vi "Watch_SPEC.vi"() -> ()   [LabVIEW 2015]
uses:
  <vilib>/Platform/TimedLoop/XDataNode/timing_clust.ctl
  <vilib>/Platform/TimedLoop/XDataNode/nitl_modes.ctl
  <vilib>/Platform/TimedLoop/XDataNode/wakeup.ctl
  <userlib>/caLab/Private/Get_PV-1D.vi
  <vilib>/platform/TimedLoop/XDataNode/XDataNode.xnode
  <vilib>/Platform/TimedLoop/XDataNode/XDNodeRunTimeDep.lvlib
panel:
  out "EPICS_PVs":string
  in  "Logbook":string(combo)
  out "subarray 2":dbl[](array[numeric])
  out "subarray":dbl[](array[numeric])
  out "XY Graph":cluster{dbl[], dbl[]}(graph)
  out "concatenated string 3":string
  out "standard error 5":string
  out "standard output 5":string
  out "File Name 5":string
  out "x = y? 3":bool
  out "standard output 4":string
  out "standard error 4":string
  out "concatenated string 2":string
  out "spreadsheet string 2":string
  in  "Filter txt":string="*.txt"
  out "File Name 4":string
  out "spreadsheet string 3":string
  out "concatenated string 6":string
  out "standard error 3":string
  out "standard output 3":string
  in  "OK Button":bool
  in  "Maindir":string="P:\\bl13-0\\bl13-2\\dt_SES100\\"
  in  "stop 2":bool
  in  "ELOG":string
  out "path":path
  in  "Subdir":string="2016\\Nilsson\\"
  out "PV Names (dup)":string[](array[string])
  out "PV2ELOG":string
  # "Set a folder to watch using the\nPath control. You can also\nset a filter for a certain type\nof file to watch for (such as\n*.bmp). Then run the\nexample. Whenever you create\na new file in that directory that\nmatches the filter, New File Name\nwill update to let you know the\nnew file name."
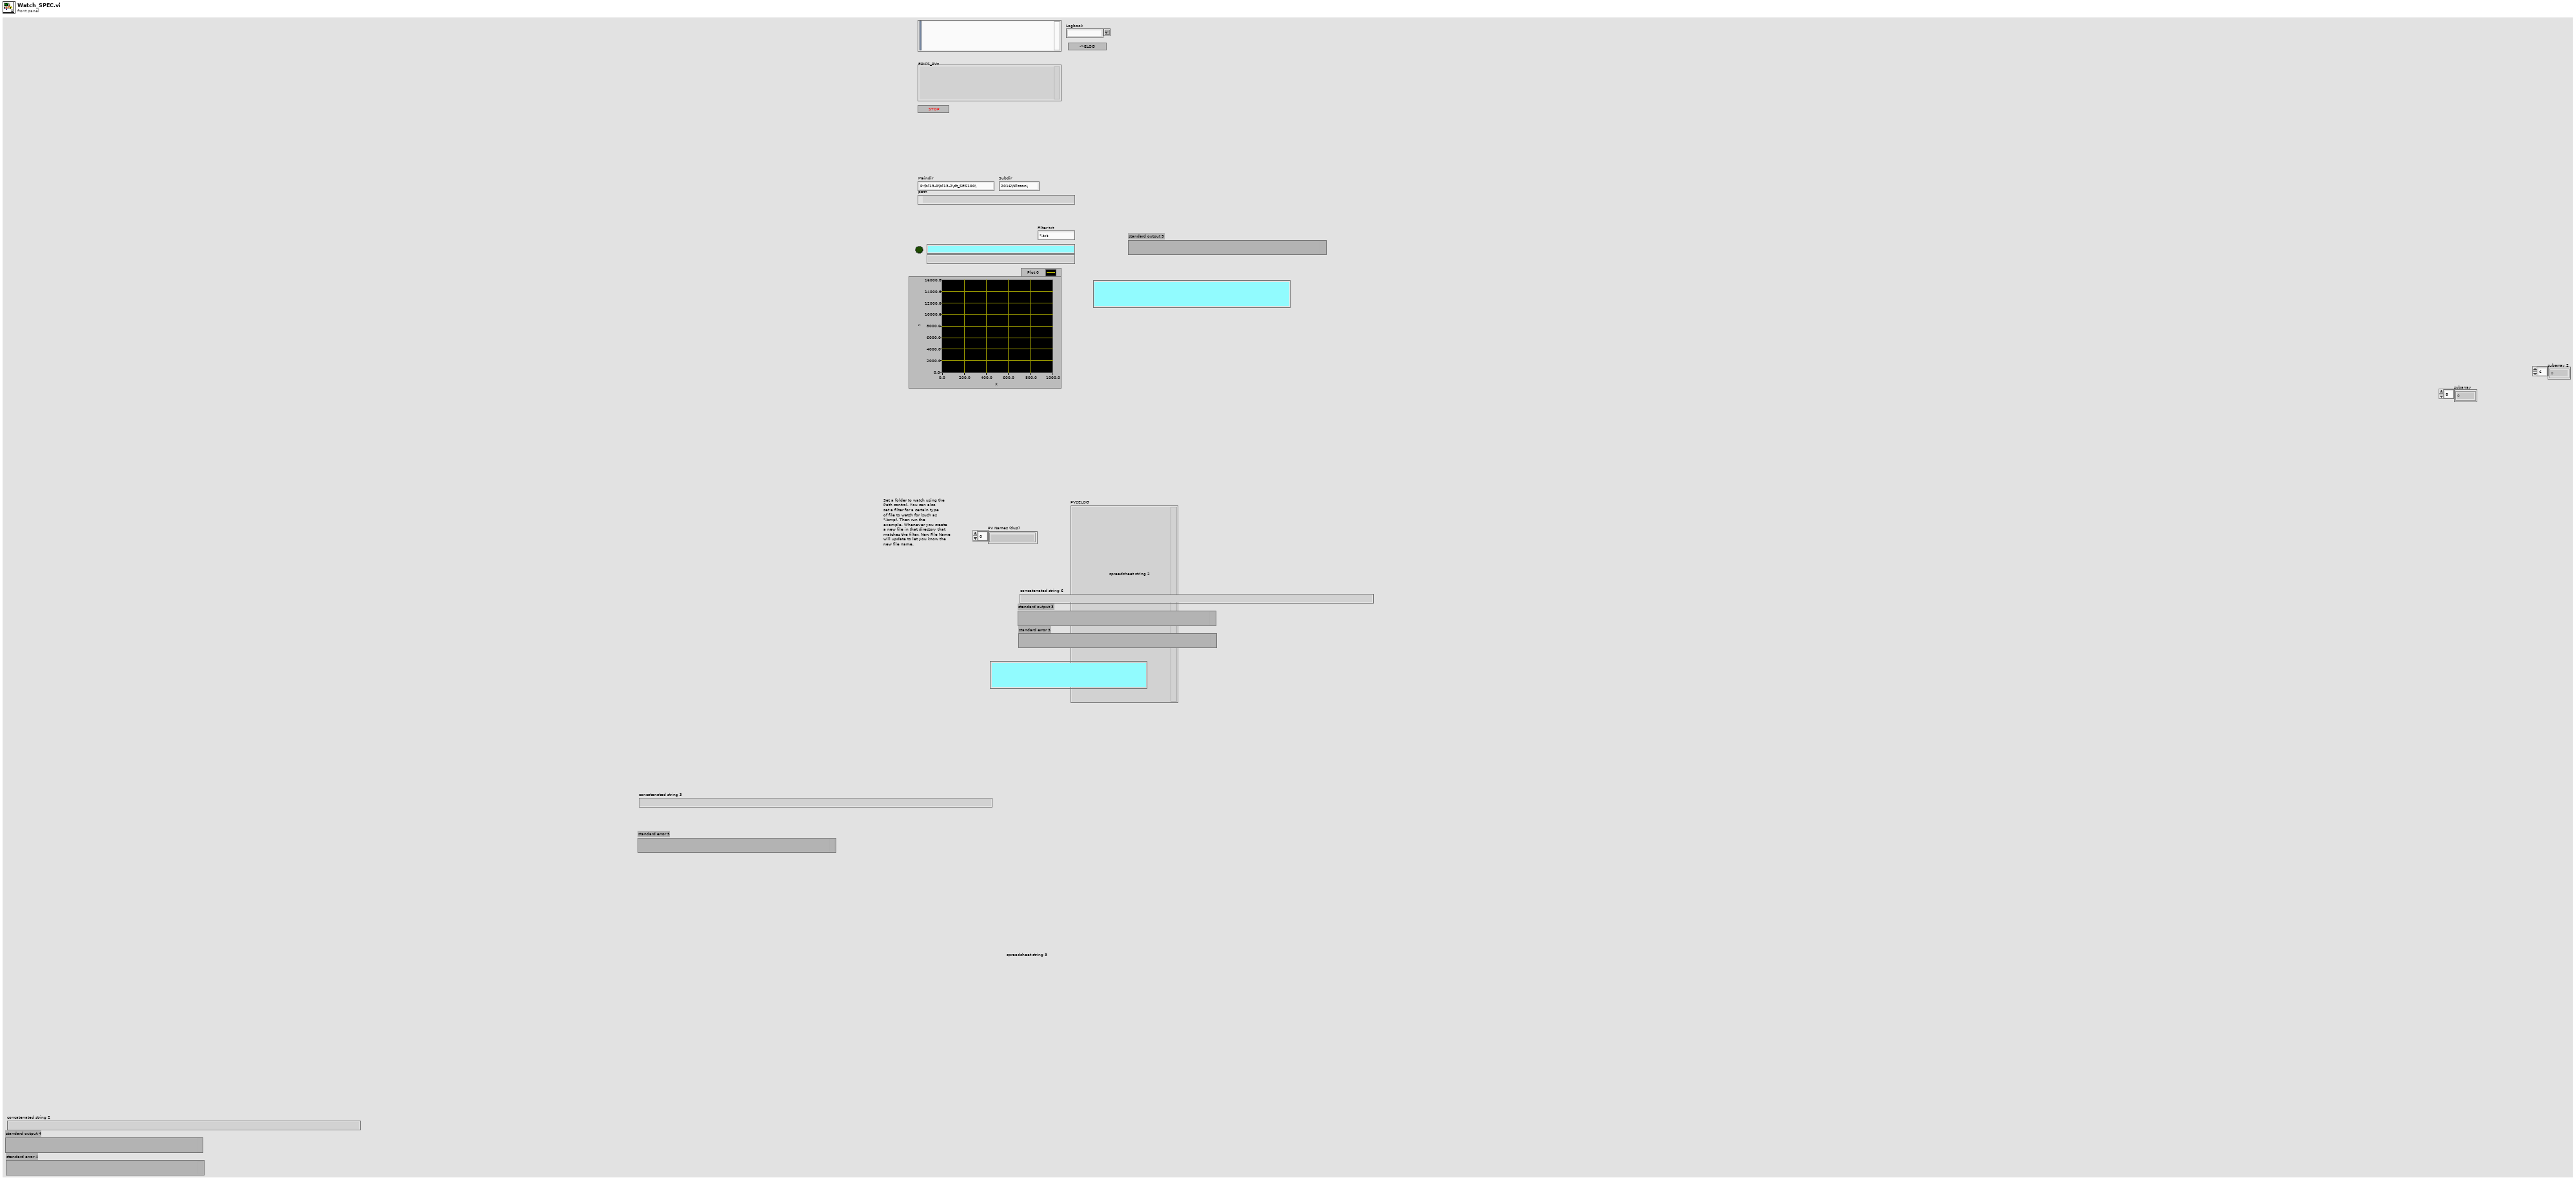
[diagram p1: front panel]
types:
  T1 = typedef "XDNodeRunTimeDep.lvlib/timing_clust.ctl" = cluster{"Expected End [f-1]":u64, "Actual End [f-1]":u64, "Finished Late? [f-1]":bool, "Expected End [i-1]":u64, "Actual End [i-1]":u64, "Finished Late? [i-1]":bool, "Expected Start [i]":u64, "Actual Start [i]":u64, "Expected Start [f]":u64, "Actual Start [f]":u64, "Source Name":string, "Structure Name":string, "Period":i64, "Deadline":i64, "Offset":i64, "Start":i64, "Priority":i32, "Timeout":i32, "Mode":T2, "Wakeup Reason":T3, "Error":errorcluster, "Source Type":string, "Secondary Source Type":string, "Global End Time":u64, "Global Start Time":u64, "Frame Duration":u64, "Iteration Duration":u64, "Assigned CPU":i32, "I/O Scan Engine Mode":u32}
  T2 = typedef "XDNodeRunTimeDep.lvlib/nitl_modes.ctl" = enum32{"No Change", "Process missed periods, maintain original phase", "Discard missed periods, maintain original phase", "Process missed periods, ignore original phase", "Discard missed periods, ignore original phase"}
  T3 = typedef "XDNodeRunTimeDep.lvlib/wakeup.ctl" = enum32{"Normal", "Aborted", "Asynchronous wakeup", "Timing source error", "Timed loop error", "Timeout"}
  T4 = enum16{"open", "replace", "create", "open or create", "replace or create", "replace or create with confirmation"}
  T5 = typedef "imagedata.ctl" = cluster{"image type":i32, "image depth":i32, "image":u8[], "mask":u8[], "colors":u32[], "Rectangle":cluster{"left":i16, "top":i16, "right":i16, "bottom":i16}}
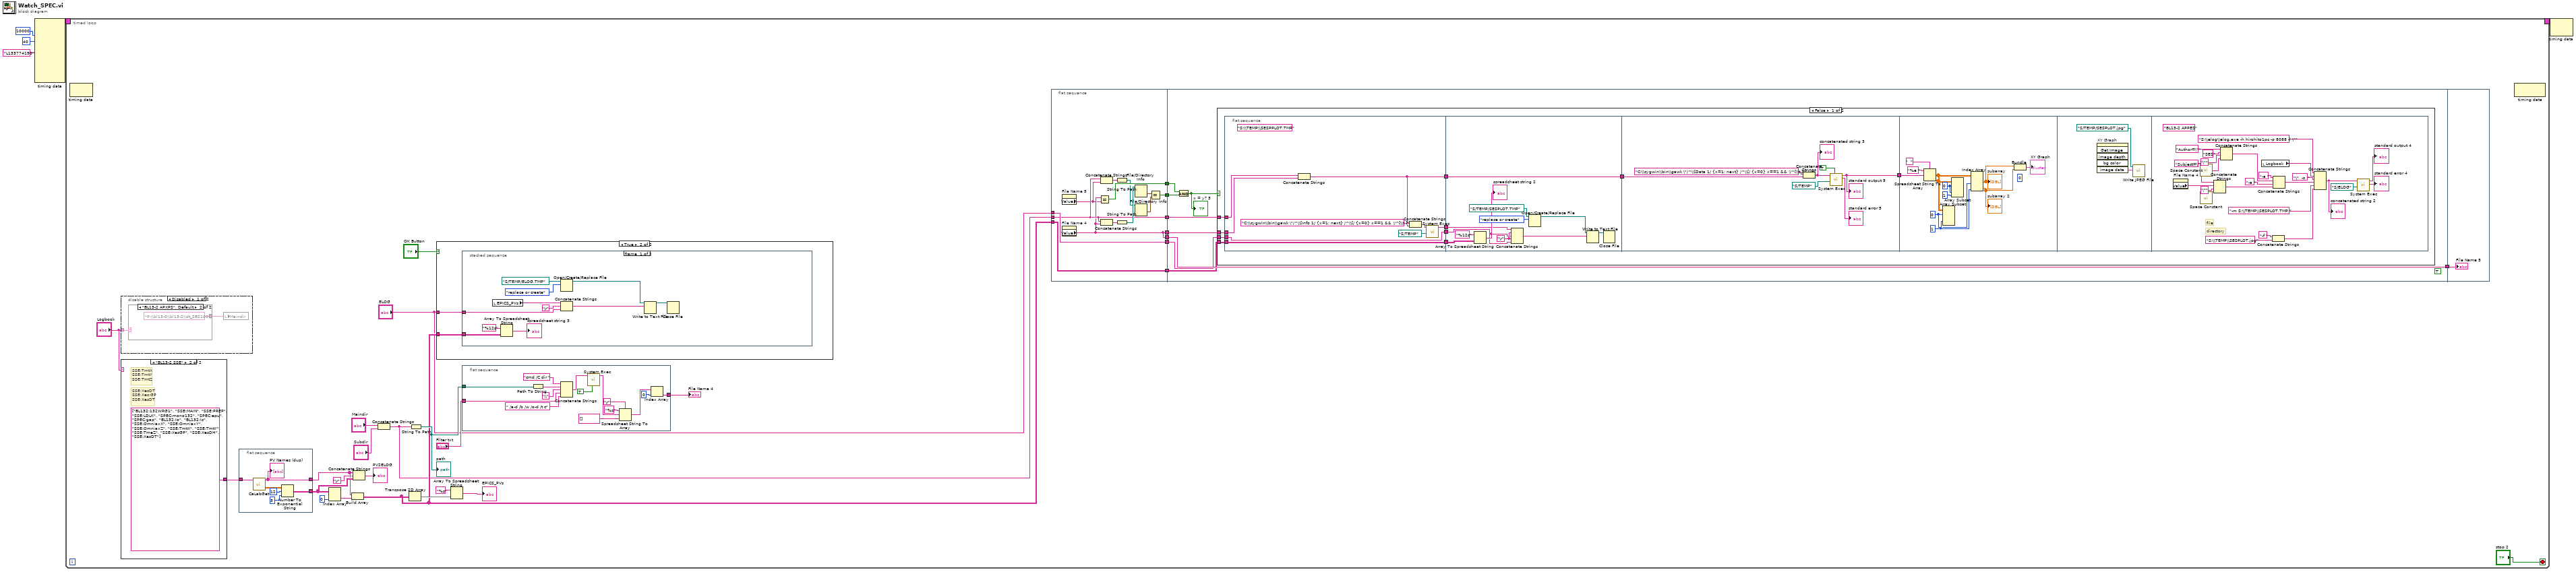
[diagram p0: block diagram]
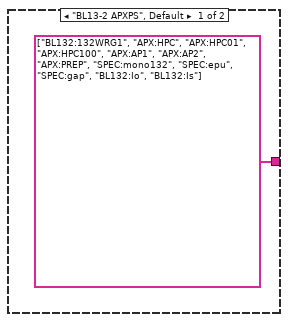
[diagram p2: hidden frame]
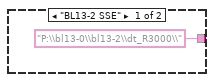
[diagram p3: hidden frame]
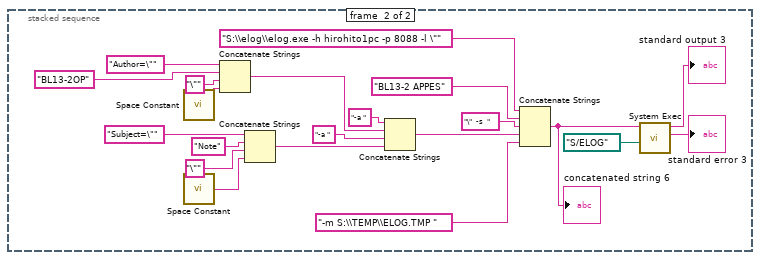
[diagram p7: hidden frame]
diagram:
  n1 = node-c288(i64 10000 ("Period"), 40 ("Priority"), "L133774190" ("Structure Name")) -> (w5:T1)  [unwired: 6 in]
  n2 = timed-loop {
    timing: w5 -> [_]
    timing-out: [_] -> w4
    stop <- "stop 2" stop-if-true
    n3 = node-c288() -> ()  [unwired: 1 in, 1 out]
    n4 = disable-structure shown="Disabled" {
      disable-tunnel: "Logbook" -> [w38 _]
      frame Disabled {
        n5 = case shown="\"BL13-2 APXPS\", Default" w38 {
          tunnel: ["P:\\bl13-0\\bl13-2\\dt_R3000\\" ("Maindir") "P:\\bl13-0\\bl13-2\\dt_SES100\\" ("Maindir")] -> w37
          frame "BL13-2 SSE" {
          }
          frame "BL13-2 APXPS", Default {
          }
        }
        n6 = local write "Maindir"(w37) -> ()
      }
      frame Enabled {
      }
    }
    n7 = case shown="\"BL13-2 SSE\"" "Logbook" {
      tunnel: [string[] ["BL132:132WRG1", "APX:HPC", "APX:HPC01", "APX:HPC100", "APX:AP1", "APX:AP2", "APX:PREP", "SPEC:mono132", "SPEC:epu", "SPEC:gap", "BL132:Io", "BL132:Is"] string[] ["BL132:132WRG1", "SSE:MAIN", "SSE:PREP", "SSE:LDLK", "SPEC:mono132", "SPEC:epu", "SPEC:gap", "BL132:Io", "BL132:Is", "SSE:OmniaxX", "SSE:OmniaxY", "SSE:OmniaxZ", "SSE:TmtX", "SSE:TmtY", "SSE:TmeZ", "SSE:XesGP", "SSE:XesDH", "SSE:XesDT"]] -> w12
      frame "BL13-2 APXPS", Default {
      }
      frame "BL13-2 SSE" {
        # "SSE:TmtX\nSSE:TmtY\nSSE:TmtZ"
        # "SSE:XesDT\nSSE:Xes:GP\nSSE:XesDT"
      }
    }
    n8 = flat-sequence {
      tunnel: [w44] -> w30
      tunnel: [w43] -> w28
      tunnel: w12 -> [w41]
      frame #0 {
        n9 = call-poly <userlib>:"CaLabGet.vi"("PV Names"=w41) -> ("PV Names (dup)"=w43:string[], "Value Array (number)"=w42:dbl[][])  [unwired: 8 in, 5 out]
        "PV Names (dup)" <- w43
        n10 = Number To Exponential String(number=w42, precision (6)=i16 3, 3:i16 12 ("width (-)")) -> (E-format string=w44:string[][])  [unwired: 1 in]
      }
    }
    n11 = Index Array(array=w30, index (col)=0) -> (element=w31:string[])  [unwired: 1 in]
    n12 = Build Array "Build Array"(w28, w31) -> (w8:string[][])
    n13 = Concatenate Strings(w28, "\r", w30) -> (→"PV2ELOG":string)
    n14 = Concatenate Strings("Maindir", "Subdir") -> (w7:string)
    n15 = Transpose 2D Array(2D array=w8) -> (transposed array=w11:string[][])
    n16 = String To Path(string=w7) -> (path=w22:path)
    "path" <- w22
    n17 = case shown="True" "OK Button" {
      tunnel: "ELOG" -> [_ w160]
      tunnel: w8 -> [_ w159]
      frame False {
      }
      frame True {
        n18 = stacked-sequence {
          tunnel: w160 -> [w164 _]
          tunnel: w159 -> [w163 _]
          frame #0 {
            n19 = local read "EPICS_PVs"() -> (w162:string)
            n20 = Array To Spreadsheet String(array=w163, 3:"%12s" ("format string")) -> (spreadsheet string=→"spreadsheet string 3":string)  [unwired: 1 in]
            n21 = Open/Create/Replace File(file path (use dialog)=path "S:/TEMP/ELOG.TMP", operation (0:open)=T4."replace or create") -> (refnum out=w171:refnum<file>)  [unwired: 4 in, 2 out]
            n22 = Concatenate Strings(w162, "\r", w164) -> (w165:string)
            n23 = Write to Text File(file (use dialog)=w171, text=w165) -> (refnum out=w170:refnum<file>)  [unwired: 2 in, 2 out]
            n24 = Close File(refnum=w170) -> ()  [unwired: 1 in, 2 out]
          }
          frame #1 {
            n25 = call <vilib>:"Space Constant.vi"() -> ("String"=w178:string)
            n26 = call <vilib>:"Space Constant.vi"() -> ("String"=w179:string)
            n27 = Concatenate Strings("Author=\"" ("string"), "BL13-2OP", "\"" ("string"), w178) -> (w176:string)
            n28 = Concatenate Strings("Subject=\"" ("string"), "Note" ("string"), "\"" ("string"), w179) -> (w174:string)
            n29 = Concatenate Strings("-a ", w176, "-a " ("string"), w174) -> (w175:string)
            n30 = Concatenate Strings("S:\\elog\\elog.exe -h hirohito1pc -p 8088 -l \"" ("command line"), "BL13-2 APPES", "\"  -s  " ("command line"), w175, "-m S:\\TEMP\\ELOG.TMP " ("string")) -> (w187:string)
            "concatenated string 6" <- w187
            n31 = call <vilib>:"System Exec.vi"("working directory"=path "S:/ELOG", "command line"=w187) -> ("standard error"=→"standard error 3":string, "standard output"=→"standard output 3":string)  [unwired: 6 in, 2 out]
          }
        }
      }
    }
    n32 = Array To Spreadsheet String(array=w11, 3:"%s" ("format string")) -> (spreadsheet string=→"EPICS_PVs":string)  [unwired: 1 in]
    n33 = flat-sequence {
      tunnel: w22 -> [w150]
      tunnel: [w147] -> w24
      tunnel: "Filter txt" -> [w145]
      frame #0 {
        n34 = Path To String(path=w150) -> (string=w153:string)
        n35 = Concatenate Strings("cmd /C dir " ("command line"), w153, "\\" ("string"), w145, " /a-d /b /w /o-d /t c" ("command line")) -> (w151:string)
        n36 = call <vilib>:"System Exec.vi"("run minimized? (F)"=TRUE, "command line"=w151) -> ("standard output"=w157:string)  [unwired: 4 in, 5 out]
        n37 = Spreadsheet String To Array(delimiter (Tab)="\r", format string="%s", spreadsheet string=w157, array type (2D Dbl)=string[] []) -> (array=w149:string[])
        n38 = Index Array(array=w149, index=0) -> (element=w147:string)
      }
    }
    n39 = flat-sequence {
      tunnel: [w53] -> w21
      tunnel: [w59] -> w20
      tunnel: [w54] -> w18
      tunnel: [w53] -> w17
      tunnel: [w58] -> w16
      tunnel: w7 -> [w54]
      tunnel: "ELOG" -> [w58]
      tunnel: w8 -> [w57]
      tunnel: [w57] -> w15
      tunnel: [w47] -> w14
      tunnel: w21 -> [w67]
      tunnel: [w67] -> w19
      tunnel: w20 -> [w61]
      tunnel: w18 -> [w66]
      tunnel: w17 -> [w65]
      tunnel: w16 -> [w64]
      tunnel: w15 -> [w63]
      tunnel: w14 -> [w62]
      tunnel: w19 -> [w143]
      frame #0 {
        n40 = property on="File Name 5" class="Str"() -> ("Value"=w52:string)  [unwired: 2 in, 2 out]
        n41 = property on="File Name 4" class="Str"() -> ("Value"=w53:string)  [unwired: 2 in, 2 out]
        n42 = Equal?(x=w53, y=w52) -> (x = y?=w59:bool)
        n43 = Concatenate Strings(w54, w52) -> (w51:string)
        n44 = Concatenate Strings(w54, w53) -> (w50:string)
        n45 = String To Path(string=w51) -> (path=w55:path)
        n46 = String To Path(string=w50) -> (path=w56:path)
        n47 = File/Directory Info(path=w56) -> (last mod=w49:timestamp)  [unwired: 1 in, 6 out]
        n48 = File/Directory Info(path=w55) -> (last mod=w48:timestamp)  [unwired: 1 in, 6 out]
        n49 = Equal?(x=w49, y=w48) -> (x = y?=w47:bool)
      }
      frame #1 {
        (unwired) TRUE
        n50 = And(x=w61, y=w62) -> (x .and. y?=w60:bool)
        "x = y? 3" <- w60
        n51 = case shown="False" w60 {
          tunnel: w63 -> [w77 _]
          tunnel: w64 -> [w76 _]
          tunnel: w66 -> [w75 _]
          tunnel: w65 -> [w74 _]
          frame False {
            n52 = flat-sequence {
              tunnel: w76 -> [w80]
              tunnel: w77 -> [w78]
              tunnel: w75 -> [w83]
              tunnel: w74 -> [w82]
              tunnel: [w81] -> w72
              tunnel: [w80] -> w70
              tunnel: [w79] -> w69
              tunnel: [w78] -> w68
              tunnel: w72 -> [w98]
              tunnel: [w98] -> w71
              tunnel: w70 -> [w89]
              tunnel: w69 -> [w88]
              tunnel: w68 -> [w87]
              tunnel: w71 -> [w101]
              tunnel: [w99] -> w73
              tunnel: w73 -> [w106]
              frame #0 {
                (unwired) "S:\\TEMP\\SESPPLOT.TMP" ("string")
                n53 = Concatenate Strings(w83, w82) -> (w81:string)
                n54 = Concatenate Strings("C:\\cygwin\\bin\\gawk \"/^\\[Info 1/ {x=1; next} /^\\[/ {x=0} x==1 && !/^[\\t ]*$/\" " ("command line"), w81) -> (w84:string)
                n55 = call <vilib>:"System Exec.vi"("working directory"=path "S:/TEMP", "command line"=w84) -> ("standard output"=w79:string)  [unwired: 6 in, 3 out]
              }
              frame #1 {
                w96 = "\r"
                n56 = Array To Spreadsheet String(array=w87, 3:"%12s" ("format string")) -> (spreadsheet string=w94:string)  [unwired: 1 in]
                "spreadsheet string 2" <- w94
                n57 = Concatenate Strings(w88, w96, w94, w96, w89) -> (w95:string)
                n58 = Open/Create/Replace File(file path (use dialog)=path "S:/TEMP/SESPLOT.TMP", operation (0:open)=T4."replace or create") -> (refnum out=w97:refnum<file>)  [unwired: 4 in, 2 out]
                n59 = Write to Text File(file (use dialog)=w97, text=w95) -> (refnum out=w90:refnum<file>)  [unwired: 2 in, 2 out]
                n60 = Close File(refnum=w90) -> ()  [unwired: 1 in, 2 out]
              }
              frame #2 {
                n61 = Concatenate Strings("C:\\cygwin\\bin\\gawk \"/^\\[Data 1/ {x=1; next} /^\\[/ {x=0} x==1 && !/^[\\t ]*$/\" " ("command line"), w101) -> (w105:string)
                "concatenated string 3" <- w105
                n62 = call <vilib>:"System Exec.vi"("wait until completion? (T)"=TRUE, "working directory"=path "S:/TEMP", "command line"=w105) -> ("standard error"=→"standard error 5":string, "standard output"=w99:string)  [unwired: 5 in, 2 out]
                "standard output 5" <- w99
              }
              frame #3 {
                (unwired) 0 ("index")
                w111 = 1 ("index")
                w110 = 0 ("index")
                w114 = 0 ("index")
                n63 = Spreadsheet String To Array(delimiter (Tab)="  " ("format string"), format string="%e ", spreadsheet string=w106) -> (array=w112:dbl[][])  [unwired: 1 in]
                n64 = Array Subset(array=w112, index (row)=w110, index (col)=w111) -> ()  [unwired: 2 in, 1 out]
                n65 = Array Subset(array=w112, index (row)=w114, index (col)=w114, length (col)=1 ("index")) -> ()  [unwired: 1 in, 1 out]
                n66 = Index Array(array=w112, index (col) #1=w110, index (col) #2=w111) -> (element #1=w109:dbl[], element #2=w108:dbl[])  [unwired: 2 in]
                "subarray" <- w109
                "subarray 2" <- w108
                n67 = Bundle(w109, w108) -> (→"XY Graph":cluster{dbl[], dbl[]})  [unwired: 1 in]
              }
              frame #4 {
                n68 = invoke on="XY Graph" class="XYGraph (strict)" method="Get Image"() -> ("image data"=w117:T5)  [unwired: 6 in, 5 out]
                n69 = call <vilib>:"Write JPEG File.vi"("image data"=w117, "path to JPEG file"=path "S:/TEMP/SESPLOT.jpg" ("file path (use dialog)")) -> ()  [unwired: 8 in, 2 out]
              }
              frame #5 {
                (unwired) "BL13-2 APPES"
                # "file"
                # "directory"
                n70 = property on="File Name 4" class="Str"() -> ("Value"=w123:string)  [unwired: 2 in, 2 out]
                n71 = call <vilib>:"Space Constant.vi"() -> ("String"=w129:string)
                n72 = call <vilib>:"Space Constant.vi"() -> ("String"=w130:string)
                n73 = Concatenate Strings("Subject=\"" ("string"), w123, "\"" ("string"), w130) -> (w125:string)
                n74 = Concatenate Strings("Author=\"" ("string"), "SES", "\"" ("string"), w129) -> (w127:string)
                n75 = local read "Logbook"() -> (w119:string)
                n76 = Concatenate Strings("-f " ("string"), "S:\\TEMP\\SESPLOT.jpg" ("string")) -> (w121:string)
                n77 = Concatenate Strings("-a ", w127, "-a " ("string"), w125) -> (w126:string)
                n78 = Concatenate Strings("S:\\elog\\elog.exe -h hirohito1pc -p 8088 -l \"" ("command line"), w119, "\"  -s  " ("command line"), w126, "-m S:\\TEMP\\SESPLOT.TMP " ("string"), w121) -> (w138:string)
                "concatenated string 2" <- w138
                n79 = call <vilib>:"System Exec.vi"("working directory"=path "S:/ELOG", "command line"=w138) -> ("standard error"=→"standard error 4":string, "standard output"=→"standard output 4":string)  [unwired: 6 in, 2 out]
              }
            }
          }
          frame True {
          }
        }
      }
      frame #2 {
        "File Name 5" <- w143
      }
    }
    n80 = node-c288() -> ()  [unwired: 1 in, 1 out]
    "File Name 4" <- w24
  }
  n81 = node-c288(w4) -> ()  [unwired: 1 out]
